vi "calc_phase_map.vi"(4 "ul_ar_pxar_input_pxarray":u16[][][](array[numeric]), 5 "String":string="fringe") -> (1 "phase map":T1(plugin-control))   [LabVIEW 2011]
uses:
  global_vars.vi
  <vilib>/express/express arith-compare/Formula/XNode/ExpressFormulaBlockNode.xnode
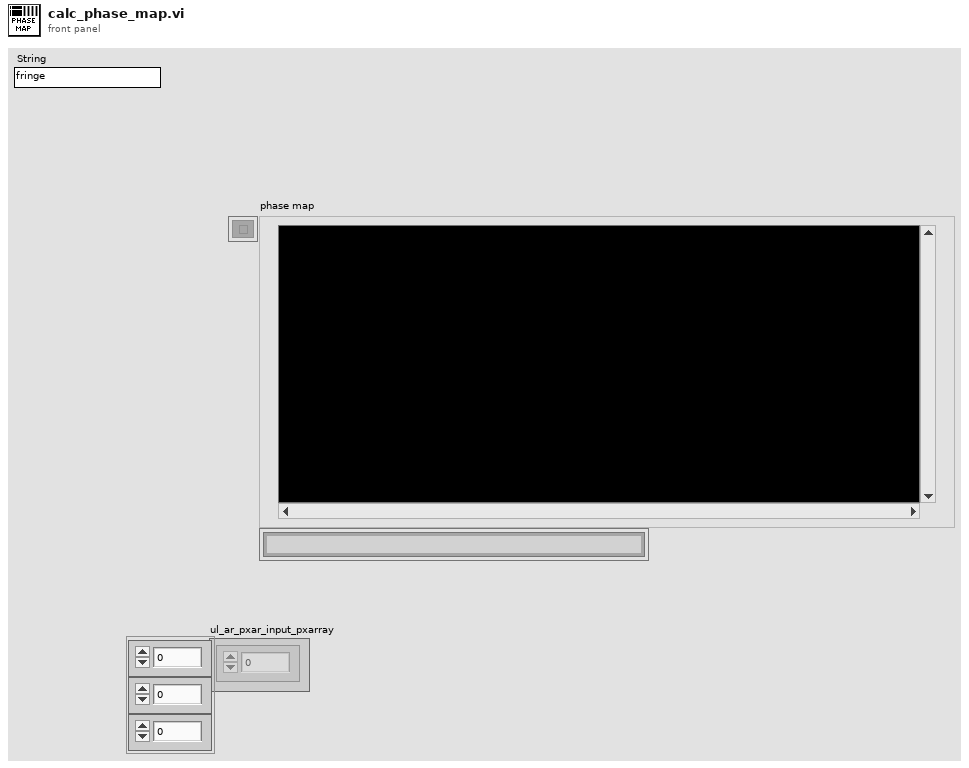
[diagram p1: front panel]
types:
  T1 = typedef "IMAQ Image.ctl" = refnum<image>
  T2 = typedef "Image Type" = u32
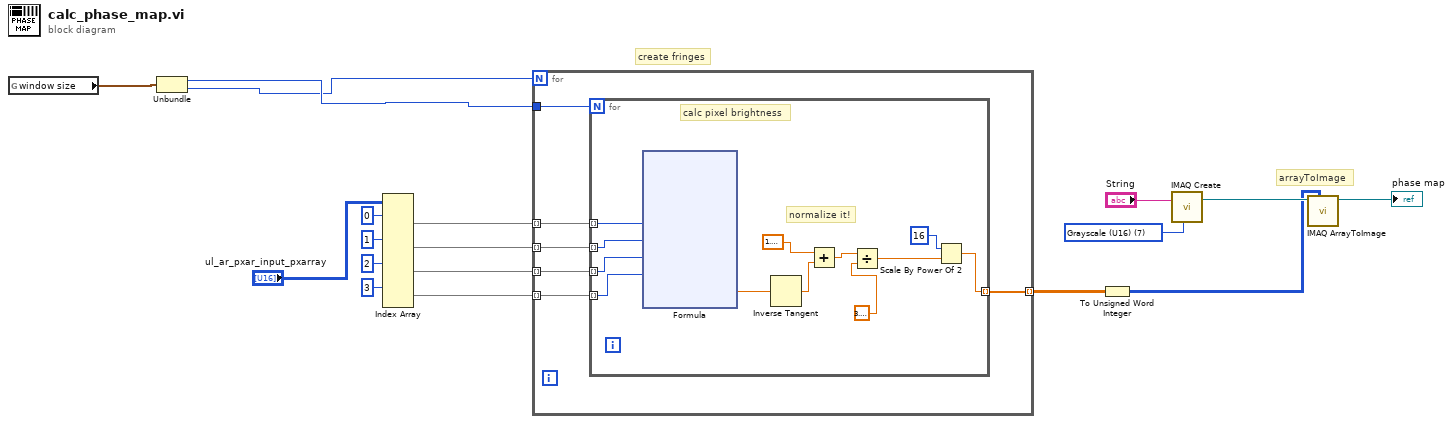
[diagram p0: block diagram]
diagram:
  w13 = T2 7 items=["Grayscale (U8)", "Grayscale (I16)", "Grayscale (SGL)", "Complex (CSG)", "RGB (U32)", "HSL (U32)", "RGB (U64)", "Grayscale (U16)"] ("Image Type")
  # "create fringes"
  # "arrayToImage"
  n1 = global read "global_vars.vi" "window size"() -> (w12:cluster{"x Width(Px)":i32, "y height(Px)":i32})
  n2 = Unbundle(w12) -> ("x Width(Px)"=w16:i32, "y height(Px)"=w15:i32)
  n3 = Index Array(array="ul_ar_pxar_input_pxarray", index (dim 0) #1=0 ("index (page)"), index (dim 0) #2=1 ("index (page)"), index (dim 0) #3=2 ("index (page)"), index (dim 0) #4=3 ("index (page)")) -> (element #1=w6:u16[][], element #2=w5:u16[][], element #3=w4:u16[][], element #4=w3:u16[][])  [unwired: 8 in]
  n4 = for {
    N: w15 -> [_]
    tunnel: w16 -> [w24]
    tunnel: w6 -> [w23] mode=indexing
    tunnel: w5 -> [w22] mode=indexing
    tunnel: w4 -> [w21] mode=indexing
    tunnel: w3 -> [w20] mode=indexing
    tunnel: [w19] -> w2 mode=indexing
    n5 = for {
      N: w24 -> [_]
      tunnel: w23 -> [w36] mode=indexing
      tunnel: w22 -> [w35] mode=indexing
      tunnel: w21 -> [w34] mode=indexing
      tunnel: w20 -> [w33] mode=indexing
      tunnel: [w30] -> w19 mode=indexing
      # "normalize it!"
      # "calc pixel brightness"
      n6 = xnode ("Formula")("A1"=w36, "A2"=w35, "A3"=w34, "A4"=w33) -> ("Result"=w32:dbl)  [unwired: 1 in, 1 out]
      n7 = Inverse Tangent(1:w32) -> (0:w29:dbl)
      n8 = Add(x=1.5707963267948966, y=w29) -> (x+y=w27:dbl)
      n9 = Divide(x=w27, y=3.141592653589793) -> (x/y=w25:dbl)
      n10 = Scale By Power Of 2(n=16, x=w25) -> (x*2^n=w30:dbl)
    }
  }
  n11 = To Unsigned Word Integer(number=w2) -> (unsigned 16bit integer=w1:u16[][])
  n12 = call "IMAQ Create"("Image Name"="String", "Image Type"=w13) -> ("New Image"=w14:T1)  [unwired: 2 in, 2 out]
  n13 = call "IMAQ ArrayToImage"("Image Pixels (U16)"=w1, "Image"=w14) -> ("Image Out"=→"phase map":T1)  [unwired: 8 in, 1 out]
